vi "STM Read Meta Data (Serial Ref).vi"(6 "Options":T3={"Ignore Timeout Error"=TRUE, "timeout ms (1000)"=1000}, 8 "error in":errorcluster, 11 "VISA resource name":refnum<visa-resource-name>) -> (0 "error out":errorcluster, 1 "Meta data":T2[](array[typedef]), 3 "Connection Info Out":T1)   [LabVIEW 2010]
doc: "This VI reads the meta data information from a remote computer. Use this VI to retrieve the variable names and types that a remote computer exports.\n\nThis VI parses the data and returns a cluster containing the meta data information.\n\nCopyright 2015, 2016, 2017 National Instruments Corporation\n\nLicensed under the Apache License, Version 2.0 (the \"License\"); you may not use this file except in compliance with the License.\n\n You may obtain a copy of the License at\n\n http://www.apache.org/licenses/LICENSE-2.0\n\nUnless required by applicable law or agreed to in writing, software distributed under the License is distributed on an \"AS IS\" BASIS, WITHOUT WARRANTIES OR CONDITIONS OF ANY KIND, either express or implied.\n\nSee the License for the specific language governing permissions and limitations under the License."
uses:
  stm_MetaDataElement.ctl
  stm_Serial Read Options.ctl
  stm_Serial Connection Info.ctl
  Serial/Read Meta Data (Serial Clst).vi
  NI STM.lvlib
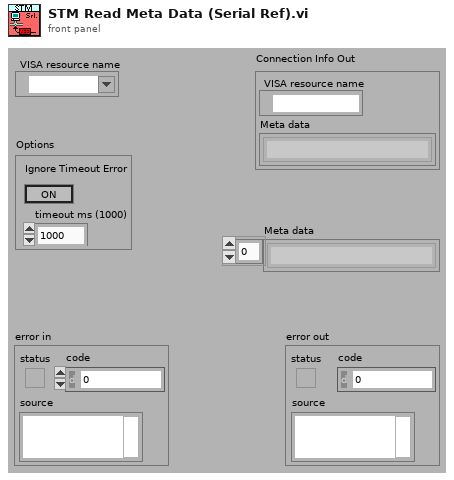
[diagram p1: front panel]
types:
  T1 = typedef "stm_Serial Connection Info.ctl" = cluster{"VISA resource name":refnum<visa-resource-name>, "Meta data":T2[]}
  T2 = typedef "stm_MetaDataElement.ctl" = string
  T3 = typedef "stm_Serial Read Options.ctl" = cluster{"Ignore Timeout Error":bool, "timeout ms (1000)":u32}
  T4 = typedef "NI STM.lvlib/MetaDataElement.ctl" = string
  T5 = typedef "NI STM.lvlib/Serial Connection Info.ctl" = cluster{"VISA resource name":refnum<visa-resource-name>, "meta data":T4[]}
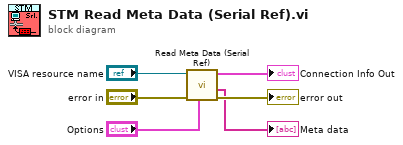
[diagram p0: block diagram]
diagram:
  n1 = call "Read Meta Data (Serial Ref).vi"("options"="Options", "error in"="error in", "VISA resource name"="VISA resource name") -> ("error out"=→"error out":errorcluster, "meta data"=→"Meta data":T4[], "connection info out"=→"Connection Info Out":T5)  [unwired: 6 in]
